vi "Write Show Overlay.vi"(8 "error in (no error)":errorcluster, 10 "Overlay?":bool, 11 "Analyze BaseClass in":refnum<class "Analyze BaseClass.lvclass">) -> (0 "error out":errorcluster, 3 "Analyze BaseClass out":refnum<class "Analyze BaseClass.lvclass">)   [LabVIEW 2020, in "Analyze.lvlib" / "Analyze BaseClass.lvclass"]
uses:
  Analyze BaseClass.lvclass
  Analyze BaseClass.lvclass/Analyze BaseClass.ctl
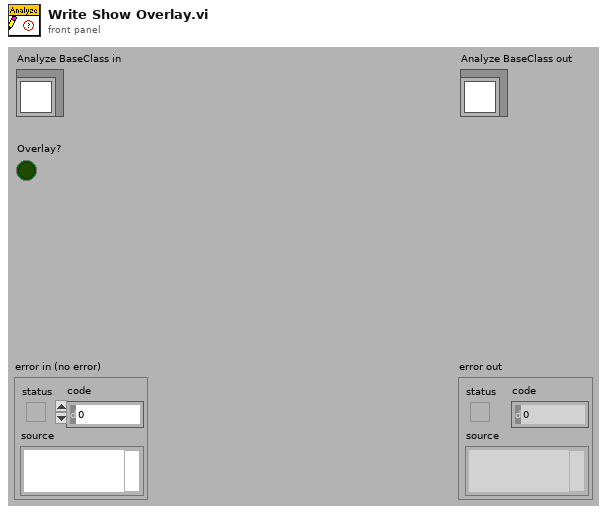
[diagram p1: front panel]
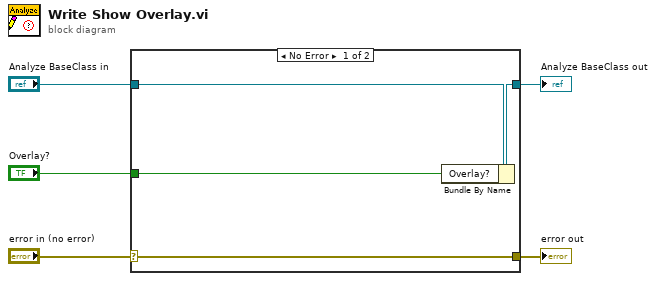
[diagram p0: block diagram]
diagram:
  n1 = case shown="No Error" "error in (no error)" {
    selector: "error in (no error)" -> [w9 w10]
    tunnel: [w9 w10] -> w4
    tunnel: [w7 w11] -> w2
    tunnel: "Analyze BaseClass in" -> [w8 w11]
    tunnel: "Overlay?" -> [w6 _]
    frame No Error {
      n2 = Bundle By Name(cluster=w8, "Overlay?"=w6) -> (w7:refnum<class "Analyze BaseClass.lvclass">)
    }
    frame Error {
    }
  }
  "error out" <- w4
  "Analyze BaseClass out" <- w2
